vi "DetPort2.vi"() -> ()   [LabVIEW 2013]
uses:
  SystemCode/SysControl/Slot.ctl
  <vilib>/Utility/error.llb/Error Cluster From Error Code.vi
  GlobalValue.vi
  <vilib>/ErrorRing/Error Ring.xnode
panel:
  out "检测结果":string
  out "数值":i32
  in  "DET":bool
  out "Port":string[](array[string])
  in  "退出":bool
  out "error out":errorcluster caption="错误输出"
  in  "error in (no error)":errorcluster caption="错误输入（无错误）"
  # "1.插好连接线\n2.左侧和右侧测试工位放入并连接好T-BOX待测品。\n3.点击下面按钮等待检测通信接口完成。"
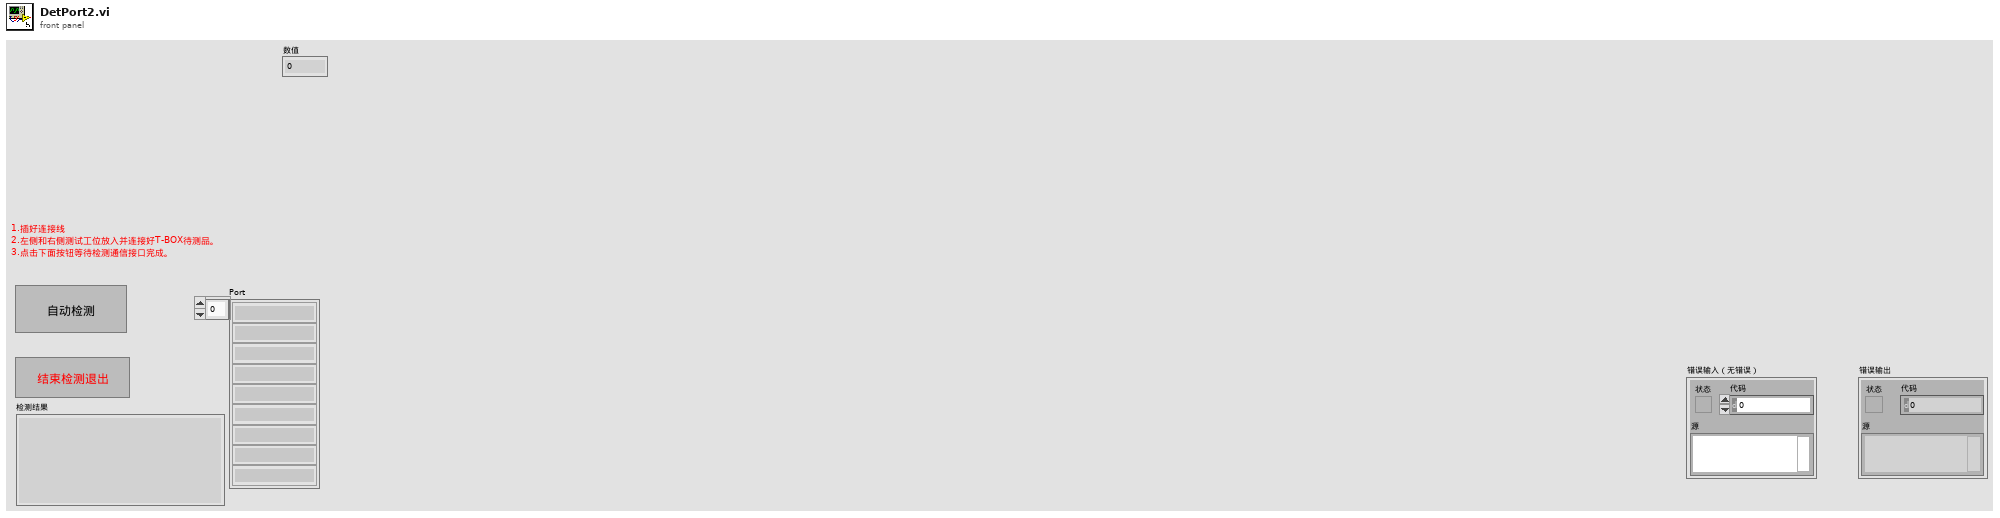
[diagram p1: front panel]
types:
  T1 = typedef "Slot.ctl" = enum16{"Slot1", "Slot2", "Slot3", "Slot4"}
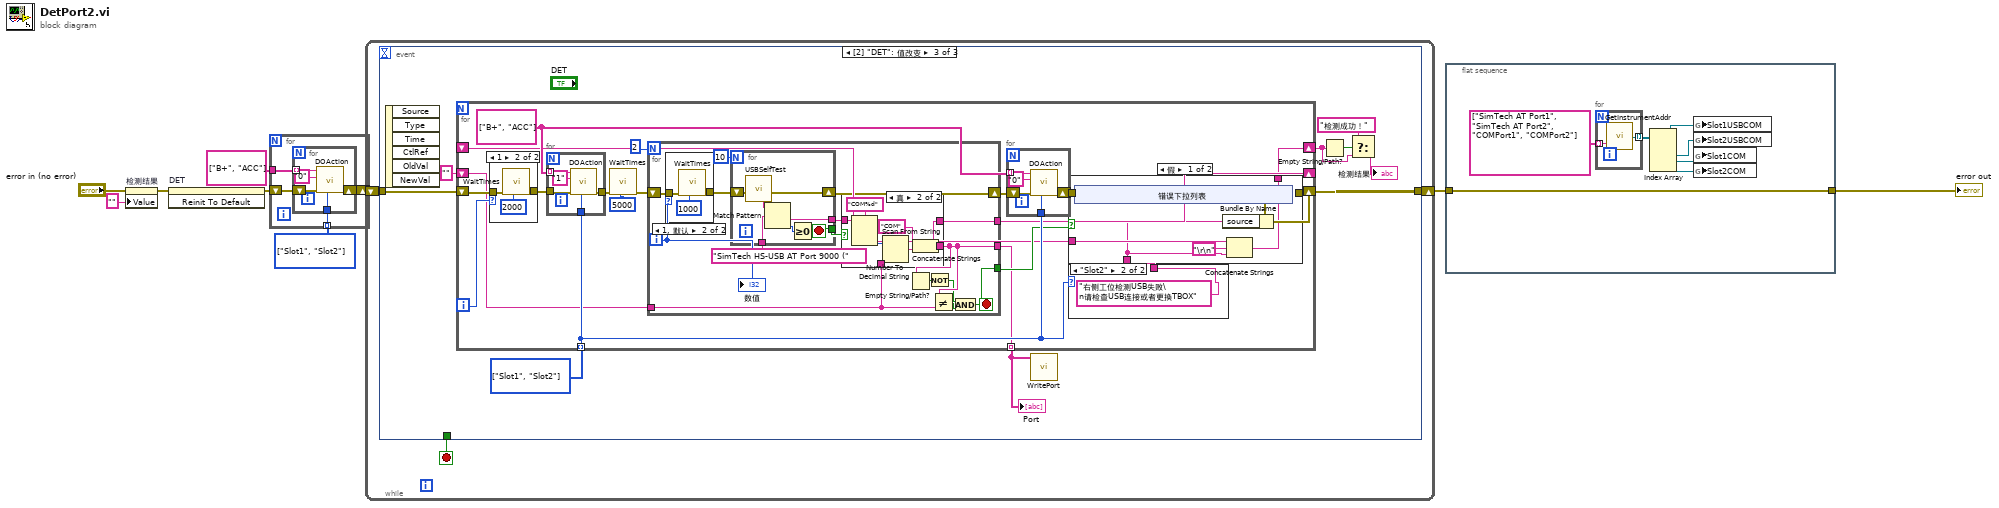
[diagram p0: block diagram]
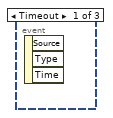
[diagram p2: hidden frame]
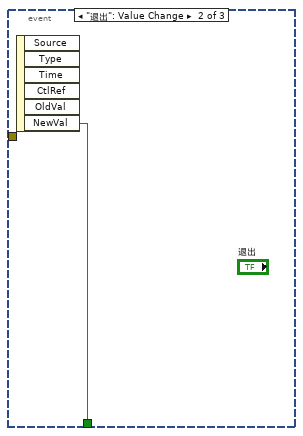
[diagram p3: hidden frame]
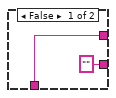
[diagram p5: hidden frame]
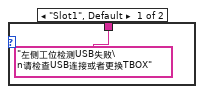
[diagram p7: hidden frame]
diagram:
  w7 = T1[] [enum."Slot1", enum."Slot2"] items=["Slot1", "Slot2", "Slot3", "Slot4"]
  n1 = property on="检测结果" class="Str"(error in="error in (no error)", "Value"="" ("检测结果")) -> (error out=w1:errorcluster)  [unwired: 1 in, 1 out]
  n2 = invoke on="DET" class="Bool" method="Reinit To Default"(error in=w1) -> (error out=w6:errorcluster)  [unwired: 2 in, 2 out]
  n3 = for {
    tunnel: string[] ["B+", "ACC"] -> [w13]
    tunnel: w7 -> [w12] mode=indexing
    shift-right: [w10] -> w5
    shift-left: w6 -> [w11]
    n4 = for {
      tunnel: w12 -> [w18]
      tunnel: w13 -> [w17] mode=indexing
      shift-right: [w14] -> w10
      shift-left: w11 -> [w15]
      n5 = call "DOAction.vi"("Slot"=w18, "error in"=w15, "State"="0", "CH"=w17) -> ("error out"=w14:errorcluster)  [unwired: 7 in]
    }
  }
  n6 = while {
    shift-right: [w19] -> w9
    shift-left: w5 -> [w20]
    stop <- w21 stop-if-true
    n7 = event shown="[2] \"DET\": 值改变" {
      selector: _ -> [_ _ _]
      dyn-events: _ -> [_ _ _]
      timeout: _ -> [_ _ _]
      tunnel: [_ w22 _] -> w21
      tunnel: w20 -> [_ _ w29]
      tunnel: [_ _ w30] -> w19
      event Timeout {
        n8 = event-data() -> ()  [unwired: 1 in, 3 out]
      }
      event "退出": Value Change {
        n9 = event-data() -> ("NewVal"=w22:bool)  [unwired: 1 in, 5 out]
      }
      event "DET": Value Change {
        w31 = T1[] [enum."Slot1", enum."Slot2"] items=["Slot1", "Slot2", "Slot3", "Slot4"]
        n10 = event-data() -> ()  [unwired: 1 in, 6 out]
        n11 = for {
          shift-right: [w42] -> w30
          shift-left: w29 -> [w39]
          tunnel: w31 -> [w46] mode=indexing
          tunnel: [w37] -> w28 mode=indexing
          shift-right: [w34] -> _
          shift-left: "" -> [w36]
          shift-right: [w32] -> w23
          shift-left: _ -> [w33]
          i -> [w40]
          w47 = string[] ["B+", "ACC"]
          n12 = case shown="1" w40 {
            tunnel: w39 -> [w85 w87]
            tunnel: [w85 w86] -> w38
            frame 0, Default {
            }
            frame 1 {
              n13 = call "WaitTimes.vi"("WaitTimes"=u32 2000, "error in (no error)"=w87) -> ("error out"=w86:errorcluster)  [unwired: 9 in]
            }
          }
          n14 = for {
            tunnel: w46 -> [w112]
            tunnel: w47 -> [w111] mode=indexing
            tunnel: w38 -> [w109]
            tunnel: [w108] -> w50
            n15 = call "DOAction.vi"("Slot"=w112, "error in"=w109, "State"="1", "CH"=w111) -> ("error out"=w108:errorcluster)  [unwired: 7 in]
          }
          n16 = call "WaitTimes.vi"("WaitTimes"=u32 5000, "error in (no error)"=w50) -> ("error out"=w41:errorcluster)  [unwired: 9 in]
          n17 = for {
            N: 2 -> [_]
            tunnel: [w58] -> w37
            tunnel: [w54] -> w45
            tunnel: w36 -> [w60]
            shift-right: [w62] -> w48
            shift-left: w41 -> [w53]
            tunnel: [w59] -> w34
            i -> [w51]
            stop <- w54 stop-if-true
            n18 = case shown="1, 默认" w51 {
              tunnel: w53 -> [w66 w68]
              tunnel: [w66 w67] -> w52
              frame 0 {
              }
              frame 1, Default {
                n19 = call "WaitTimes.vi"("WaitTimes"=u32 1000, "error in (no error)"=w68) -> ("error out"=w67:errorcluster)  [unwired: 9 in]
              }
            }
            n20 = for {
              N: 10 -> [_]
              tunnel: [w82] -> w64
              tunnel: "SimTech HS-USB AT Port 9000 (" ("正则表达式") -> [w81]
              shift-right: [w80] -> w62
              shift-left: w52 -> [w84]
              tunnel: [w79] -> w61
              stop <- w79 stop-if-true
              n21 = call "USBSelfTest.vi"("error in (no error)"=w84) -> ("error out"=w80:errorcluster, "CmdOut"=w78:string)  [unwired: 8 in, 1 out]
              n22 = Match Pattern(string=w78, regular expression=w81) -> (after substring=w82:string, offset past match=w83:i32)  [unwired: 1 in, 2 out]
              n23 = Greater Or Equal To 0?(x=w83) -> (x >= 0?=w79:bool)
            }
            n24 = case shown="真" w61 {
              tunnel: w64 -> [_ w73]
              tunnel: ["" w72] -> w58
              tunnel: [w70 w72] -> w59
              tunnel: w60 -> [w70 _]
              frame False {
              }
              frame True {
                n25 = Scan From String(format string="COM%d" ("格式字符串"), input string=w73) -> (output 1=w76:i32)  [unwired: 3 in, 3 out]
                n26 = Number To Decimal String(number=w76) -> (decimal integer string=w74:string)  [unwired: 1 in]
                n27 = Concatenate Strings("COM" ("字符串"), w74) -> (w72:string)
              }
            }
            n28 = Empty String/Path?(string/path=w58) -> (empty?=w57:bool)
            n29 = Not(x=w57) -> (.not. x?=w56:bool)
            n30 = Not Equal?(x=w58, y=w60) -> (x != y?=w55:bool)
            n31 = And(x=w56, y=w55) -> (x .and. y?=w54:bool)
            "数值" <- w51
          }
          n32 = for {
            tunnel: w46 -> [w107]
            tunnel: w47 -> [w106] mode=indexing
            shift-right: [w103] -> w43
            shift-left: w48 -> [w104]
            n33 = call "DOAction.vi"("Slot"=w107, "error in"=w104, "State"="0", "CH"=w106) -> ("error out"=w103:errorcluster)  [unwired: 7 in]
          }
          n34 = case shown="\"Slot2\"" w46 {
            tunnel: ["左侧工位检测USB失败\n请检查USB连接或者更换TBOX" ("消息") "右侧工位检测USB失败\n请检查USB连接或者更换TBOX" ("消息")] -> w44
            frame "Slot1", Default {
            }
            frame "Slot2" {
            }
          }
          n35 = case shown="假" w45 {
            tunnel: [w95 w102] -> w42
            tunnel: w43 -> [_ w102]
            tunnel: w44 -> [w92 _]
            tunnel: w33 -> [w94 w101]
            tunnel: [w93 w101] -> w32
            frame False {
              n36 = xnode "错误下拉列表"() -> ("错误输出"=w96:errorcluster)
              n37 = Bundle By Name(cluster=w96, "source"=w92) -> (w95:errorcluster)
              n38 = Concatenate Strings(w94, "\r\n", w92) -> (w93:string)
            }
            frame True {
            }
          }
        }
        "Port" <- w28
        n39 = call "WritePort.vi"("Port"=w28) -> ()  [unwired: 10 in, 1 out]
        n40 = Empty String/Path?(string/path=w23) -> (empty?=w26:bool)
        n41 = Select(t="检测成功！", s=w26, f=w23) -> (s? t:f=→"检测结果":string)
      }
    }
  }
  n42 = flat-sequence {
    tunnel: w9 -> [w113]
    tunnel: [w113] -> w4
    frame #0 {
      n43 = for {
        tunnel: string[] ["SimTech AT Port1", "SimTech AT Port2", "COMPort1", "COMPort2"] -> [w121] mode=indexing
        tunnel: [w120] -> w115 mode=indexing
        n44 = call "GetInstrumentAddr.vi"("String"=w121) -> ("VISA session"=w120:refnum<visa-resource-name>)  [unwired: 1 out]
      }
      n45 = Index Array(array=w115) -> (element #1=w116:refnum<visa-resource-name>, element #2=w117:refnum<visa-resource-name>, element #3=w118:refnum<visa-resource-name>, element #4=w119:refnum<visa-resource-name>)  [unwired: 4 in]
      n46 = global write "GlobalValue.vi" "Slot1USBCOM"(w116) -> ()
      n47 = global write "GlobalValue.vi" "Slot2USBCOM"(w117) -> ()
      n48 = global write "GlobalValue.vi" "Slot1COM"(w118) -> ()
      n49 = global write "GlobalValue.vi" "Slot2COM"(w119) -> ()
    }
  }
  "error out" <- w4
